vi "Search for newest time to keep.vi"(9 "newest time to keep":u64, 11 "timestamps (incrementing)":u64[](array[numeric])) -> (1 "split index":i32, 3 "timestamps (dup)":u64[](array[numeric]))   [LabVIEW 2021, in "Ring Buffer Strict Accessor.lvlib"]
uses:
  Ring Buffer Strict Accessor.lvlib
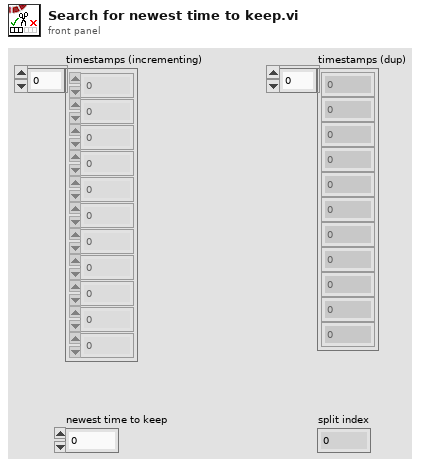
[diagram p1: front panel]
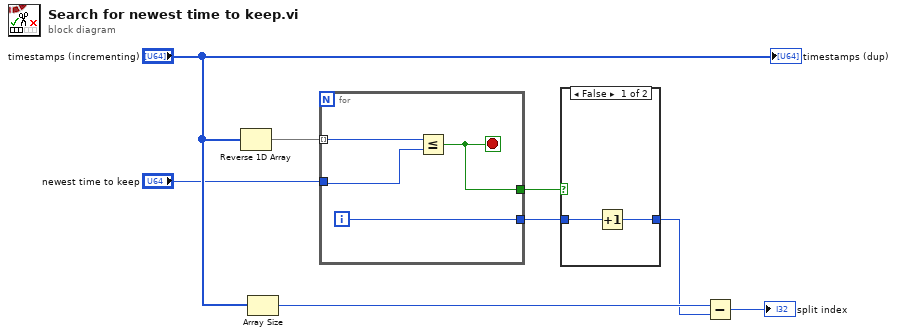
[diagram p0: block diagram]
diagram:
  n1 = Reverse 1D Array(array="timestamps (incrementing)") -> (reversed array=w8:u64[])
  n2 = Array Size(array="timestamps (incrementing)") -> (size(s)=w6:i32)
  n3 = for {
    tunnel: w8 -> [w12] mode=indexing
    tunnel: "newest time to keep" -> [w11]
    tunnel: [w10] -> w4
    tunnel: [w9] -> w5
    i -> [w10]
    stop <- w9 stop-if-true
    n4 = Less Or Equal?(x=w12, y=w11) -> (x <= y?=w9:bool)
  }
  n5 = case shown="False" w5 {
    tunnel: w4 -> [w14 w15]
    tunnel: [w13 w15] -> w3
    frame False {
      n6 = Increment(x=w14) -> (x+1=w13:i32)
    }
    frame True {
    }
  }
  n7 = Subtract(x=w6, y=w3) -> (x-y=→"split index":i32)
  "timestamps (dup)" <- "timestamps (incrementing)"
